vi "HR_to_Spreadsheet.vi"(8 "error in (no error)":errorcluster, 11 "HR Data Structure":T1) -> (0 "error out":errorcluster, 3 "HR Zones Info SpreadSheet":string)   [LabVIEW 2021]
doc: "This Vi changes Runner's data and info to speradsheet"
uses:
  Controls/HR Data Structure.ctl
  Controls/Runner's Data.ctl
  Controls/Raw Data.ctl
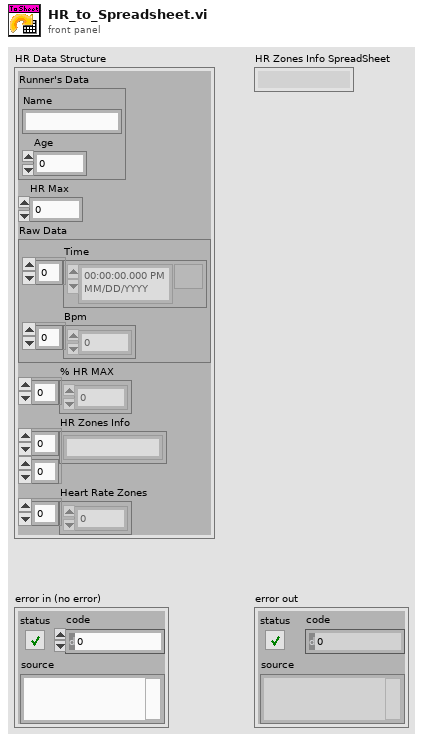
[diagram p1: front panel]
types:
  T1 = typedef "HR Data Structure.ctl" = cluster{"Runner's Data":T2, "HR Max":i32, "Raw Data":T3, "% HR MAX ":dbl[], "HR Zones Info":string[][], "Heart Rate Zones":dbl[]}
  T2 = typedef "Runner's Data.ctl" = cluster{"Name":string, "Age":i32}
  T3 = typedef "Raw Data.ctl" = cluster{"Time":timestamp[], "Bpm":i32[]}
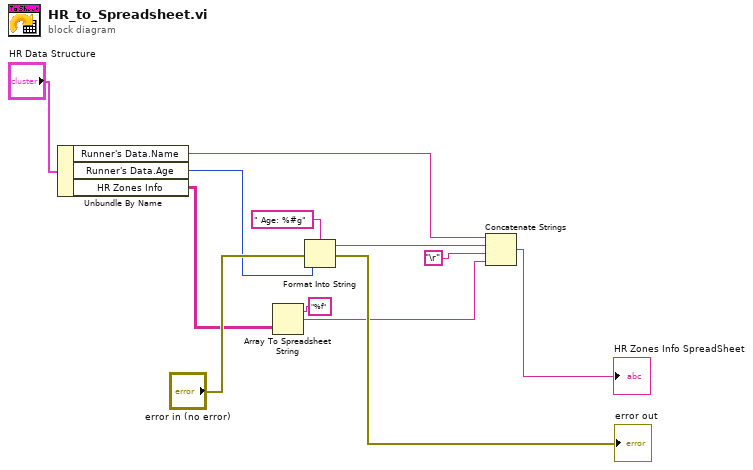
[diagram p0: block diagram]
diagram:
  n1 = Unbundle By Name("HR Data Structure") -> ("Runner's Data.Name"=w5:string, "Runner's Data.Age"=w3:i32, "HR Zones Info"=w9:string[][])
  n2 = Array To Spreadsheet String(array=w9, 3:"%f" ("format string")) -> (spreadsheet string=w10:string)  [unwired: 1 in]
  n3 = Format Into String(format string=" Age: %#g", error in="error in (no error)", w3) -> (resulting string=w6:string, error out=→"error out":errorcluster)  [unwired: 1 in]
  n4 = Concatenate Strings(w5, w6, "\r", w10) -> (→"HR Zones Info SpreadSheet":string)
